vi "Restore Build Specs After Replace.vi"(8 "error in":errorcluster, 10 "temporary project":path, 11 "custom device project":path) -> (0 "error out":errorcluster)   [LabVIEW 2020, in "Template Tool.lvlib"]
uses:
  Template Tool.lvlib
  <vilib>/xml/Load XML File.vi
  <vilib>/xml/Close Reference(Node).vi
  <vilib>/xml/NI_XML.lvlib
  <resource>/objmgr/DOMUserDefRef.rc
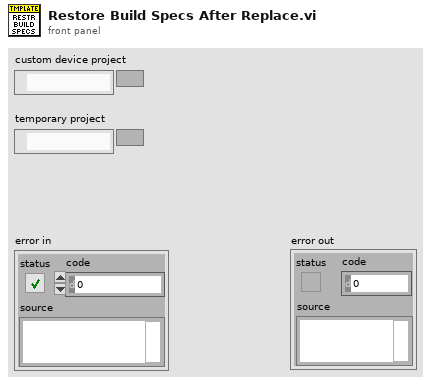
[diagram p1: front panel]
types:
  T1 = typedef "Template Tool.lvlib/Target XML Information.ctl" = cluster{"Target Name":string, "Target Node":refnum<k20>, "Build Spec Node":refnum<k20>}
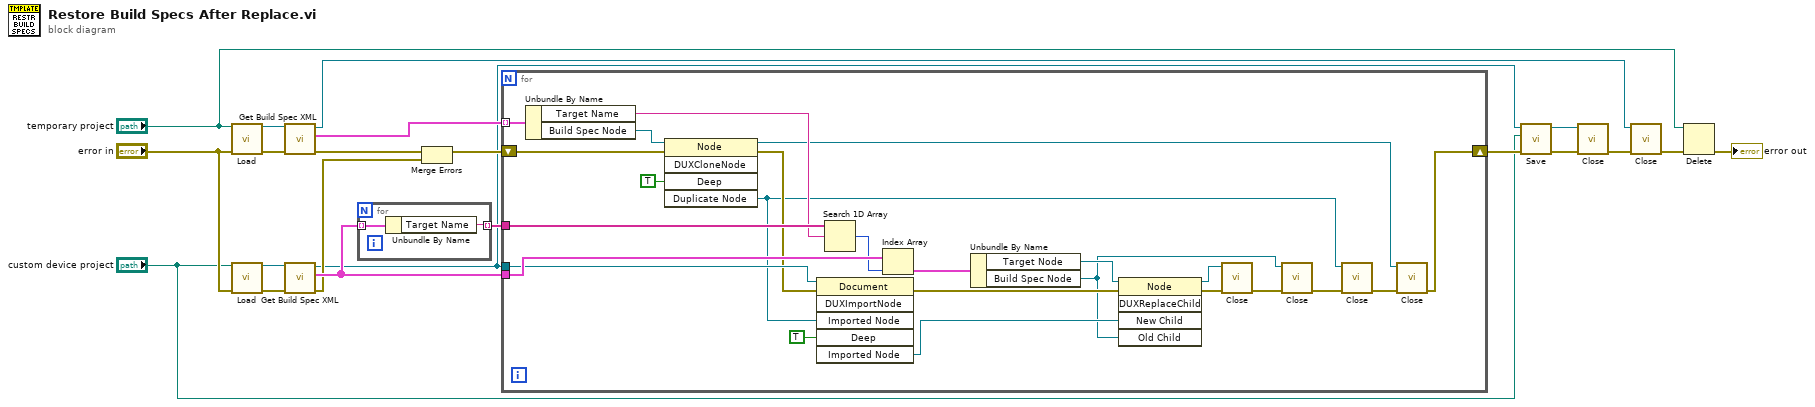
[diagram p0: block diagram]
diagram:
  n1 = call-poly <vilib>:"Load.vi"("path to XML document"="temporary project", "error in (no error)"="error in") -> ("DOM document out"=w19:refnum<k20>, "error out"=w20:errorcluster)  [unwired: 11 in, 1 out]
  n2 = call-poly <vilib>:"Load.vi"("path to XML document"="custom device project", "error in (no error)"="error in") -> ("DOM document out"=w17:refnum<k20>, "error out"=w18:errorcluster)  [unwired: 11 in, 1 out]
  n3 = call "Get Build Spec XML.vi"("error in"=w20, "DOM document"=w19) -> ("error out"=w13:errorcluster, "Build Spec XML Info"=w16:T1[], "DOM document out"=w4:refnum<k20>)  [unwired: 7 in]
  n4 = call "Get Build Spec XML.vi"("error in"=w18, "DOM document"=w17) -> ("error out"=w11:errorcluster, "Build Spec XML Info"=w15:T1[], "DOM document out"=w9:refnum<k20>)  [unwired: 7 in]
  n5 = for {
    tunnel: w15 -> [w23] mode=indexing
    tunnel: [w22] -> w14 mode=indexing
    n6 = Unbundle By Name(w23) -> ("Target Name"=w22:string)
  }
  n7 = Merge Errors(w13, w11) -> (w12:errorcluster)
  n8 = for {
    tunnel: w16 -> [w47] mode=indexing
    tunnel: w15 -> [w43]
    tunnel: w9 -> [w40]
    shift-right: [w24] -> w10
    shift-left: w12 -> [w45]
    tunnel: w14 -> [w46]
    n9 = Unbundle By Name(w47) -> ("Target Name"=w38:string, "Build Spec Node"=w39:refnum<k20>)
    n10 = invoke class="Node" method="DUXCloneNode"(reference=w39, error in=w45, "Deep"=TRUE) -> (reference out=w25:refnum<k20>, error out=w33:errorcluster, "Duplicate Node"=w27:refnum<k20>)  [unwired: 2 in, 2 out]
    n11 = invoke class="Document" method="DUXImportNode"(reference=w40, error in=w33, "Imported Node"=w27, "Deep"=TRUE) -> (error out=w37:errorcluster, "Imported Node"=w34:refnum<k20>)  [unwired: 2 in, 4 out]
    n12 = Search 1D Array(1D array=w46, element=w38) -> (index of element=w42:i32)  [unwired: 1 in]
    n13 = Index Array(array=w43, index=w42) -> (element=w36:T1)
    n14 = Unbundle By Name(w36) -> ("Target Node"=w35:refnum<k20>, "Build Spec Node"=w29:refnum<k20>)
    n15 = invoke class="Node" method="DUXReplaceChild"(reference=w35, error in=w37, "New Child"=w34, "Old Child"=w29) -> (reference out=w31:refnum<k20>, error out=w32:errorcluster)  [unwired: 1 in, 3 out]
    n16 = call-poly <vilib>:"Close.vi"("error in (no error)"=w32, "node"=w31) -> ("error out"=w30:errorcluster)  [unwired: 7 in]
    n17 = call-poly <vilib>:"Close.vi"("error in (no error)"=w30, "node"=w29) -> ("error out"=w28:errorcluster)  [unwired: 7 in]
    n18 = call-poly <vilib>:"Close.vi"("error in (no error)"=w28, "node"=w27) -> ("error out"=w26:errorcluster)  [unwired: 7 in]
    n19 = call-poly <vilib>:"Close.vi"("error in (no error)"=w26, "node"=w25) -> ("error out"=w24:errorcluster)  [unwired: 7 in]
  }
  n20 = call <vilib>:"Save.vi"("error in (no error)"=w10, "XML file path"="custom device project", "DOM document in"=w9) -> ("error out"=w7:errorcluster, "DOM document out"=w6:refnum<k20>)  [unwired: 6 in, 1 out]
  n21 = call-poly <vilib>:"Close.vi"("error in (no error)"=w7, "node"=w6) -> ("error out"=w5:errorcluster)  [unwired: 7 in]
  n22 = call-poly <vilib>:"Close.vi"("error in (no error)"=w5, "node"=w4) -> ("error out"=w3:errorcluster)  [unwired: 7 in]
  n23 = Delete(path (use dialog)="temporary project", error in=w3) -> (error out=→"error out":errorcluster)  [unwired: 3 in, 2 out]
